vi "ble_evt_attclient_group_found.vi"(8 "error in (no error)":errorcluster, 11 "COM Bluegiga in":refnum<visa-resource-name>) -> (0 "error out":errorcluster, 2 "service_info":u8[][](array[numeric]), 3 "COM Bluegiga out":refnum<visa-resource-name>)   [LabVIEW 2013]
uses:
  type_def/message_class.ctl
  type_def/message_type.ctl
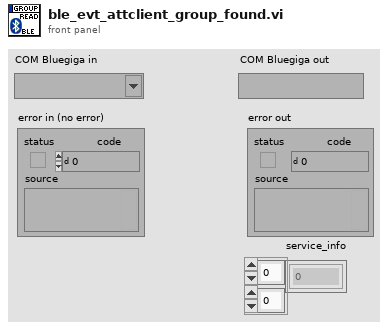
[diagram p1: front panel]
types:
  T1 = typedef "message_type.ctl" = u8
  T2 = typedef "message_class.ctl" = u8
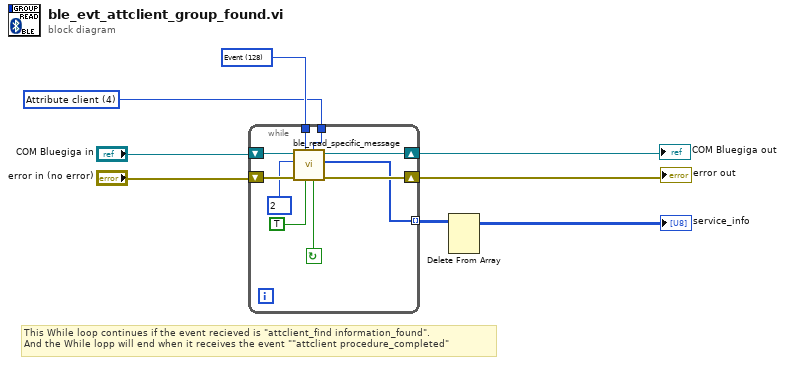
[diagram p0: block diagram]
diagram:
  w8 = T1 128 items=["Command / Response"=0, "Event"=128] ("Message Type (Response)")
  w7 = T2 4 items=["System", "Persistent Store", "Attribute database", "Connection", "Attribute client", "Security Manager", "Generic Access Profile", "Hardware"] ("Command Class (System)")
  # "This While loop continues if the event recieved is \"attclient_find information_found\".\nAnd the While lopp will end when it receives the event \"\"attclient procedure_completed\""
  n1 = while {
    tunnel: w8 -> [w18]
    tunnel: w7 -> [w14]
    shift-right: [w11] -> w6
    shift-left: "COM Bluegiga in" -> [w17]
    shift-right: [w12] -> w5
    shift-left: "error in (no error)" -> [w16]
    tunnel: [w10] -> w4 mode=indexing
    stop <- w13 continue-if-true
    n2 = call "ble_read_specific_message.vi"("Command Class (System)"=w14, "Stop if differnt to expected(F)"=TRUE, "Message Type (Response)"=w18, "error in (no error)"=w16, "Message ID (0x00)"=u8 2, "COM Bluegiga in"=w17) -> ("error out"=w12:errorcluster, "specific payload"=w10:u8[], "COM Bluegiga out"=w11:refnum<visa-resource-name>, "success?"=w13:bool)  [unwired: 1 in, 1 out]
  }
  "COM Bluegiga out" <- w6
  "error out" <- w5
  n3 = Delete From Array(array=w4) -> (array with subset deleted=→"service_info":u8[][])  [unwired: 3 in, 1 out]
